vi "RDMA - Create Rx Transfer.vi"(0 "local address":string="169.254.239.43", 5 "local port":string, 7 "rx channels":T4[](array[typedef]) {"core"."string offset" format="%d bytes"}) -> (8 "Transfer":T1={"core"={"name"="Transfer"}, "component settings"=[], "channels"=[]} {"channels"."core"."string offset" format="%d bytes"})   [LabVIEW 2023]
uses:
  Public/Documents/National Instruments/NI VeriStand 2023/Custom Devices/Data Sharing Framework/Windows/DSF Core.lvlibp/Typedefs/DSF Engine Channel Configuration.ctl
  Public/Documents/National Instruments/NI VeriStand 2023/Custom Devices/Data Sharing Framework/Windows/DSF Core.lvlibp/Typedefs/Core Channel Configuration.ctl
  Public/Documents/National Instruments/NI VeriStand 2023/Custom Devices/Data Sharing Framework/Windows/DSF Core.lvlibp/Typedefs/DSF Data Type.ctl
  Public/Documents/National Instruments/NI VeriStand 2023/Custom Devices/Data Sharing Framework/Windows/DSF Core.lvlibp/Typedefs/DSF Settings Info.ctl
  Public/Documents/National Instruments/NI VeriStand 2023/Custom Devices/Data Sharing Framework/Windows/DSF Core.lvlibp/Typedefs/DSF Engine Transfer Configuration.ctl
  Public/Documents/National Instruments/NI VeriStand 2023/Custom Devices/Data Sharing Framework/Windows/DSF Core.lvlibp/Typedefs/Core Transfer Configuration.ctl
  Public/Documents/National Instruments/NI VeriStand 2023/Custom Devices/Data Sharing Framework/Windows/DSF Core.lvlibp
  Public/Documents/National Instruments/NI VeriStand 2023/Custom Devices/Data Sharing Framework/Windows/DSF Core.lvlibp/Classes/Configuration/Core/Channel/Channel Configuration.lvclass
  Public/Documents/National Instruments/NI VeriStand 2023/Custom Devices/Data Sharing Framework/Windows/DSF Core.lvlibp/Classes/Configuration/Core/Transfer/Transfer Configuration.lvclass
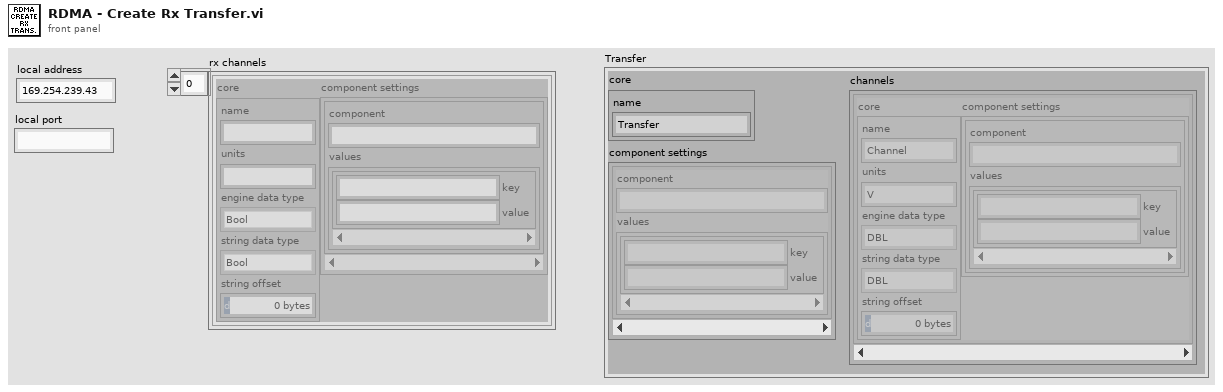
[diagram p1: front panel]
types:
  T1 = typedef "DSF Core.lvlibp/DSF Engine Transfer Configuration.ctl" = cluster{"core":T2, "component settings":T3[], "channels":T4[]}
  T2 = typedef "DSF Core.lvlibp/Transfer Configuration.lvclass/Core Transfer Configuration.ctl" = cluster{"name":string}
  T3 = typedef "DSF Core.lvlibp/DSF Settings Info.ctl" = cluster{"component":string, "values":cluster{"key":string, "value":string}[]}
  T4 = typedef "DSF Core.lvlibp/DSF Engine Channel Configuration.ctl" = cluster{"core":T5, "component settings":T3[]}
  T5 = typedef "DSF Core.lvlibp/Channel Configuration.lvclass/Core Channel Configuration.ctl" = cluster{"name":string, "units":string, "engine data type":T6, "string data type":T6, "string offset":u64}
  T6 = typedef "DSF Core.lvlibp/DSF Data Type.ctl" = enum8{"Bool", "SGL", "DBL", "I8", "I16", "I32", "I64", "U8", "U16", "U32", "U64"}
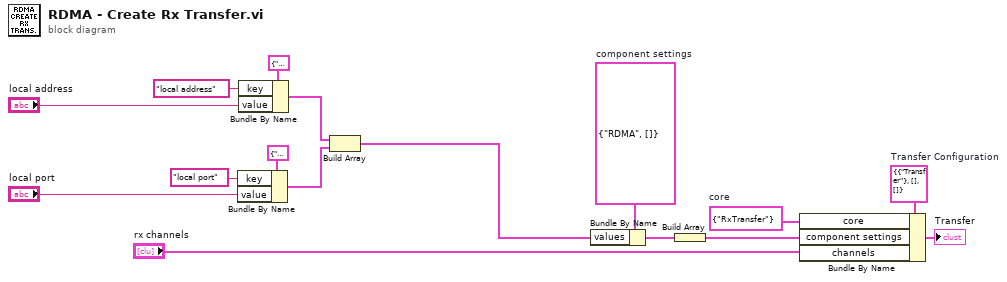
[diagram p0: block diagram]
diagram:
  w4 = T3 {"component"="RDMA", "values"=[]}  # component settings
  w5 = T2 {"name"="RxTransfer"}  # core
  w6 = T1 {"core"={"name"="Transfer"}, "component settings"=[], "channels"=[]}  # Transfer Configuration
  n1 = Bundle By Name(cluster=cluster{"key":string, "value":string} {"key"="", "value"=""} ("setting"), "key"="local port", "value"="local port") -> (w8:cluster{"key":string, "value":string})
  n2 = Bundle By Name(cluster=cluster{"key":string, "value":string} {"key"="", "value"=""} ("setting"), "key"="local address", "value"="local address") -> (w10:cluster{"key":string, "value":string})
  n3 = Build Array(w10, w8) -> (w16:cluster{"key":string, "value":string}[])
  n4 = Bundle By Name(cluster=w4, "values"=w16) -> (w3:T3)
  n5 = Build Array(w3) -> (w2:T3[])
  n6 = Bundle By Name(cluster=w6, "core"=w5, "component settings"=w2, "channels"="rx channels") -> (→"Transfer":T1)
